vi "Create Component Loader.vi"(8 "error in (no error)":errorcluster, 10 "components directory":path, 11 "Component Loader type":refnum<class "Component Loader.lvclass">) -> (0 "error out":errorcluster, 3 "Component Loader out":refnum<class "Component Loader.lvclass">)   [LabVIEW 2017, in "DSF Core.lvlib" / "Component Loader.lvclass"]
uses:
  Component Loader.lvclass
  Component Loader.lvclass/Component Loader.ctl
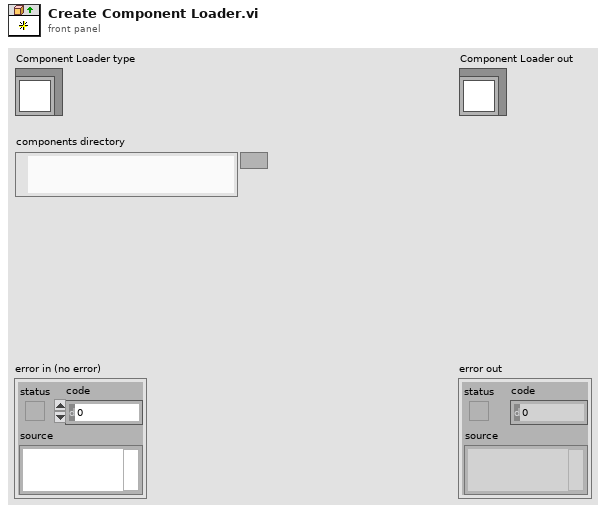
[diagram p1: front panel]
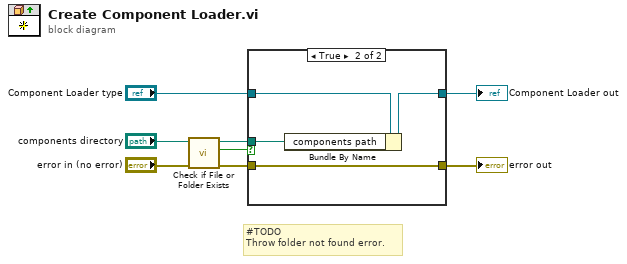
[diagram p0: block diagram]
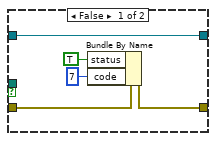
[diagram p2: hidden frame]
diagram:
  # "#TODO\nThrow folder not found error."
  n1 = call <vilib>:"Check if File or Folder Exists.vi"("error in (no error)"="error in (no error)", "path"="components directory") -> ("error out"=w3:errorcluster, "file or folder exists?"=w1:bool, "dup path"=w4:path)  [unwired: 7 in]
  n2 = case shown="True" w1 {
    tunnel: "Component Loader type" -> [w13 w17]
    tunnel: [w13 w16] -> w7
    tunnel: w4 -> [_ w15]
    tunnel: w3 -> [w12 w14]
    tunnel: [w11 w14] -> w2
    frame False {
      n3 = Bundle By Name(cluster=w12, "status"=TRUE, "code"=7) -> (w11:errorcluster)
    }
    frame True {
      n4 = Bundle By Name(cluster=w17, "components path"=w15) -> (w16:refnum<class "Component Loader.lvclass">)
    }
  }
  "error out" <- w2
  "Component Loader out" <- w7
